vi "x_2y_graph_cluster.vi"(0 "Y1":dbl, 1 "Y2":dbl, 2 "X":dbl, 3 "Chart History (10,000)":i32, 4 "Clear Graph?":bool) -> (5 "Cluster":cluster{dbl[], dbl[]})   [LabVIEW 2016]
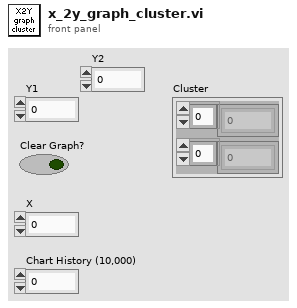
[diagram p1: front panel]
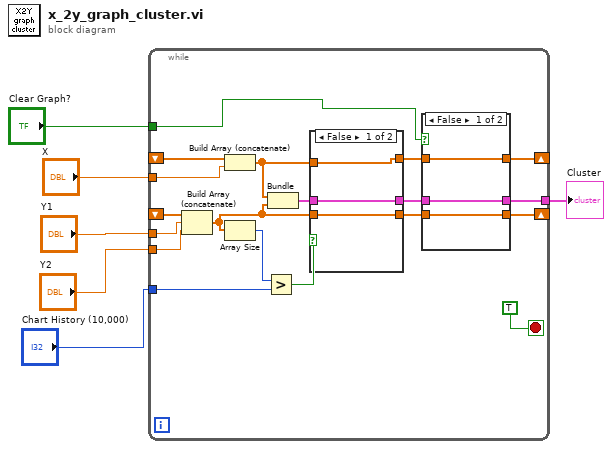
[diagram p0: block diagram]
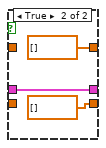
[diagram p2: hidden frame]
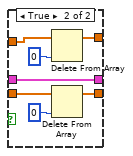
[diagram p3: hidden frame]
diagram:
  n1 = while {
    tunnel: "X" -> [w25]
    tunnel: "Y1" -> [w23]
    shift-right: [w12] -> _
    shift-left: _ -> [w24]
    shift-right: [w15] -> _
    shift-left: _ -> [w22]
    tunnel: "Chart History (10,000)" -> [w20]
    tunnel: [w10] -> w4
    tunnel: "Clear Graph?" -> [w8]
    tunnel: "Y2" -> [w7]
    stop <- TRUE stop-if-true
    n2 = Build Array (concatenate)(w22, w23, w7) -> (w17:dbl[])
    n3 = Build Array (concatenate)(w24, w25) -> (w14:dbl[])
    n4 = Array Size(array=w17) -> (size(s)=w21:i32)
    n5 = Greater?(x=w21, y=w20) -> (0:w19:bool)
    n6 = Bundle(w14, w17) -> (w18:cluster{dbl[], dbl[]})  [unwired: 1 in]
    n7 = case shown="False" w19 {
      tunnel: w18 -> [w32 w35]
      tunnel: w17 -> [w34 w37]
      tunnel: [w34 w36] -> w16
      tunnel: [w33 w40] -> w13
      tunnel: w14 -> [w33 w41]
      tunnel: [w32 w35] -> w11
      frame False {
      }
      frame True {
        n8 = Delete From Array(array=w41, index=0) -> (array with subset deleted=w40:dbl[])  [unwired: 1 in, 1 out]
        n9 = Delete From Array(array=w37, index=0) -> (array with subset deleted=w36:dbl[])  [unwired: 1 in, 1 out]
      }
    }
    n10 = case shown="False" w8 {
      tunnel: w16 -> [w28 _]
      tunnel: [w28 dbl[] []] -> w15
      tunnel: w13 -> [w27 _]
      tunnel: [w27 dbl[] []] -> w12
      tunnel: [w26 w29] -> w10
      tunnel: w11 -> [w26 w29]
      frame False {
      }
      frame True {
      }
    }
  }
  "Cluster" <- w4
